vi "SetDefaultModeValue.vi"(1 "Array in":T1[](array[typedef]) {"Modes"."Amplititute" step=0.05}, 2 "index":i32, 3 "Amplititute":dbl) -> (0 "output array":T1[](array[typedef]) {"Modes"."Amplititute" step=0.05})   [LabVIEW 2014]
uses:
  Controls/Holo Settings.ctl
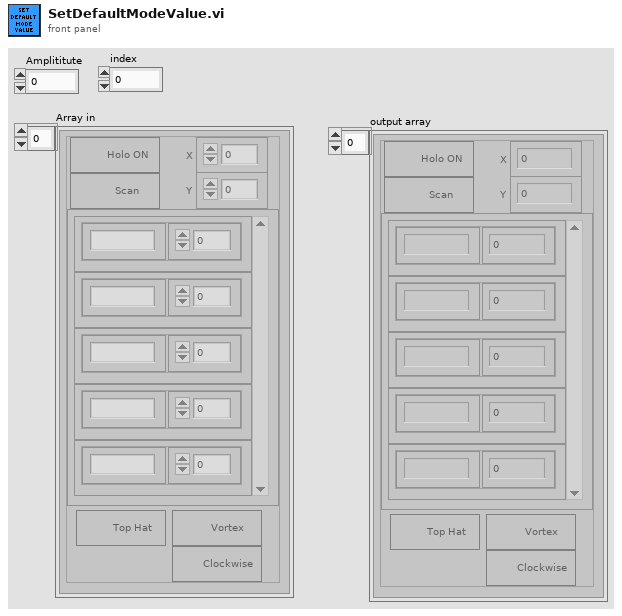
[diagram p1: front panel]
types:
  T1 = typedef "Holo Settings.ctl" = cluster{"Top Hat":bool, "Modes":cluster{"Mode ID":string, "Amplititute":dbl}[], "Vortex":bool, "Clockwise":bool, "X":dbl, "Y":dbl, "Holo ON":bool, "Scan":bool}
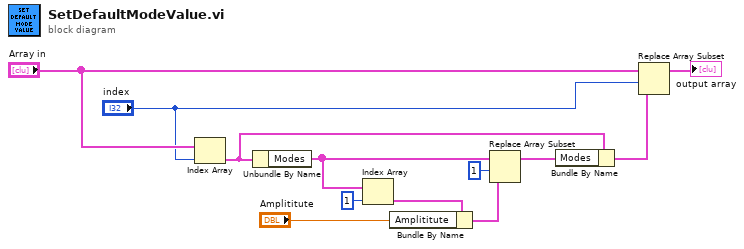
[diagram p0: block diagram]
diagram:
  n1 = Index Array(array="Array in", index="index") -> (element=w10:T1)
  n2 = Unbundle By Name(w10) -> ("Modes"=w6:cluster{"Mode ID":string, "Amplititute":dbl}[])
  n3 = Index Array(array=w6, index=1) -> (element=w4:cluster{"Mode ID":string, "Amplititute":dbl})
  n4 = Bundle By Name(cluster=w4, "Amplititute"="Amplititute") -> (w8:cluster{"Mode ID":string, "Amplititute":dbl})
  n5 = Replace Array Subset(array=w6, new element=w8, index=1) -> (w11:cluster{"Mode ID":string, "Amplititute":dbl}[])
  n6 = Bundle By Name(cluster=w10, "Modes"=w11) -> (w12:T1)
  n7 = Replace Array Subset(array="Array in", new element=w12, index="index") -> (→"output array":T1[])
